vi "5.vi"() -> ()   [LabVIEW 2017]
panel:
  out "数组":string[][](array[string])
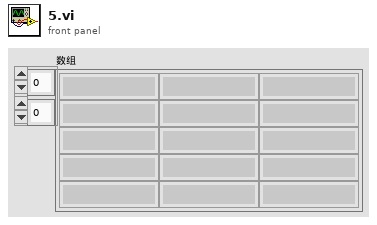
[diagram p1: front panel]
types:
  T1 = enum16{"open", "replace", "create", "open or create", "replace or create", "replace or create with confirmation"}
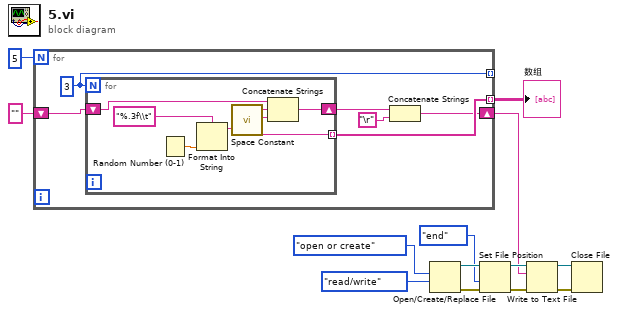
[diagram p0: block diagram]
diagram:
  n1 = for {
    N: 5 -> [_]
    tunnel: [w19] -> w8 mode=indexing
    tunnel: [w18] -> _ mode=indexing
    shift-right: [w14] -> w1
    shift-left: "" -> [w17]
    w18 = 3
    n2 = for {
      N: w18 -> [_]
      tunnel: [w21] -> w19 mode=indexing
      shift-right: [w23] -> w15
      shift-left: w17 -> [w22]
      n3 = Random Number (0-1)() -> (number: 0 to 1=w25:dbl)
      n4 = Format Into String(format string="%.3f\\t" ("格式字符串"), w25) -> (resulting string=w21:string)  [unwired: 2 in, 1 out]
      n5 = call <vilib>:"Space Constant.vi"() -> ("String"=w20:string)
      n6 = Concatenate Strings(w22, w21, w20) -> (w23:string)
    }
    n7 = Concatenate Strings(w15, "\r") -> (w14:string)
  }
  "数组" <- w8
  n8 = Open/Create/Replace File(operation (0:open)=T1."open or create" ("操作(0:open)"), access (0:read/write)=enum16{"read/write", "read-only", "write-only"}."read/write" ("权限(0:read/write)")) -> (refnum out=w13:refnum<file>, error out=w11:errorcluster)  [unwired: 4 in, 1 out]
  n9 = Set File Position(refnum=w13, from (0:start)=enum16{"start", "end", "current"}."end" ("自（0:起始）"), error in=w11) -> (refnum out=w6:refnum<file>, error out=w7:errorcluster)  [unwired: 1 in]
  n10 = Write to Text File(file (use dialog)=w6, text=w1, error in=w7) -> (refnum out=w4:refnum<file>, error out=w5:errorcluster)  [unwired: 1 in, 1 out]
  n11 = Close File(refnum=w4, error in=w5) -> ()  [unwired: 2 out]
